vi "readText.vi"(8 "error in (no error)":errorcluster, 11 "MS-Excel in":refnum<class "MS-Excel.lvclass">) -> (0 "error out":errorcluster, 2 "Text":string, 3 "MS-Excel out":refnum<class "MS-Excel.lvclass">)   [LabVIEW 2017, in "LabVIEW NPOI.lvlib" / "MS-Excel.lvclass"]
uses:
  MS-Excel.lvclass
  MS-Excel.lvclass/MS-Excel.ctl
  C:/Users/Neo/Desktop/Dev_Tools_BR/LabVIEW_NPOI/src/lib/NPOI 2.1.1/NPOI.dll
  lib/NPOI 2.1.1/NPOI.dll
  C:/Users/Neo/Desktop/Dev_Tools_BR/LabVIEW_NPOI/src/lib/NPOI 2.1.1/NPOI.OOXML.dll
  lib/NPOI 2.1.1/NPOI.OOXML.dll
  Support/File Stream/File Stream.lvlib
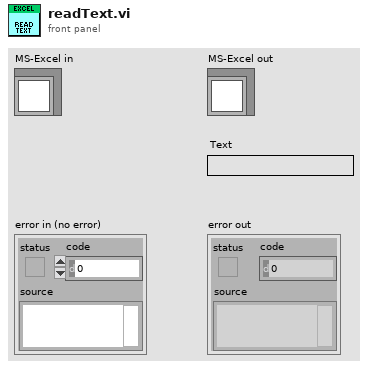
[diagram p1: front panel]
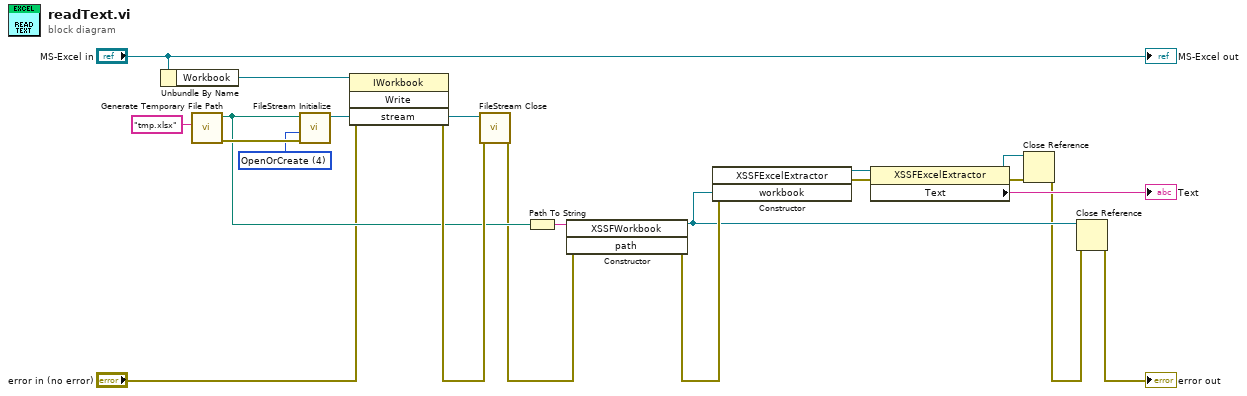
[diagram p0: block diagram]
diagram:
  w15 = 4 items=["CreateNew"=1, "Create"=2, "Open"=3, "OpenOrCreate"=4, "Truncate"=5, "Append"=6] ("mode")
  n1 = Unbundle By Name("MS-Excel in") -> ("Workbook"=w14:refnum<k24>)
  n2 = call <vilib>:"Generate Temporary File Path.vi"("Temporary File Extension (tmp)"="tmp.xlsx") -> ("error out"=w16:errorcluster, "Unique Temporary File Path"=w11:path)  [unwired: 9 in]
  n3 = call "FileStream Initialize.vi"("error in (no error)"=w16, "mode"=w15, "path"=w11) -> ("new reference"=w13:refnum<k24>)  [unwired: 7 in, 1 out]
  n4 = invoke class="IWorkbook" method="Write"(reference=w14, error in="error in (no error)", "stream"=w13) -> (error out=w12:errorcluster)  [unwired: 1 in, 3 out]
  n5 = call "FileStream Close.vi"("error in (no error)"=w12, "reference"=w13) -> ("error out"=w9:errorcluster)  [unwired: 9 in]
  n6 = Path To String(path=w11) -> (string=w10:string)
  n7 = constructor class="XSSFWorkbook"(error in=w9, "path"=w10) -> (reference out=w3:refnum<k24>, error out=w8:errorcluster)  [unwired: 2 in, 2 out]
  n8 = constructor class="XSSFExcelExtractor"(error in=w8, "workbook"=w3) -> (reference out=w18:refnum<k24>, error out=w19:errorcluster)  [unwired: 2 in, 2 out]
  n9 = property class="XSSFExcelExtractor"(reference=w18, error in=w19) -> (reference out=w4:refnum<k24>, error out=w5:errorcluster, "Text"=→"Text":string)
  n10 = Close Reference(reference=w4, error in (no error)=w5) -> (error out=w2:errorcluster)
  n11 = Close Reference(reference=w3, error in (no error)=w2) -> (error out=→"error out":errorcluster)
  "MS-Excel out" <- "MS-Excel in"
